vi "校准信息改变发送 (子VI).vi"(8 "错误输入":errorcluster caption="错误输出") -> (0 "错误输出":errorcluster)   [LabVIEW 2016, in "数据传输系统-04.lvlib"]
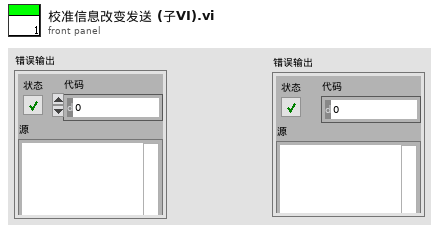
[diagram p1: front panel]
types:
  T1 = cluster{"低标液1浓度":dbl, "低标液1信号值":dbl, "低标液1启用":u16, "低标液2浓度":dbl, "低标液2信号值":dbl, "低标液2启用":u16, "低标液3浓度":dbl, "低标液3信号值":dbl, "低标液3启用":u16, "低标液4浓度":dbl, "低标液4信号值":dbl, "低标液4启用":u16, "低标液5浓度":dbl, "低标液5信号值":dbl, "低标液5启用":u16, "高标液1浓度":dbl, "高标液1信号值":dbl, "高标液1启用":u16, "高标液2浓度":dbl, "高标液2信号值":dbl, "高标液2启用":u16, "高标液3浓度":dbl, "高标液3信号值":dbl, "高标液3启用":u16, "高标液4浓度":dbl, "高标液4信号值":dbl, "高标液4启用":u16, "高标液5浓度":dbl, "高标液5信号值":dbl, "高标液5启用":u16, "低斜率":dbl, "低截距":dbl, "低二次多项式系数":dbl, "低线性相关系数":dbl, "高斜率":dbl, "高截距":dbl, "高二次多项式系数":dbl, "高线性相关系数":dbl}
  T2 = cluster{"CODMn校准信息":bool, "氨氮校准信息":bool, "总磷校准信息":bool, "总氮校准信息":bool, "CODCr校准信息":bool}
  T3 = cluster{"低标液1浓度":dbl, "低标液1信号值":dbl, "低标液1启用":u16, "低标液2浓度":dbl, "低标液2信号值":dbl, "低标液2启用":u16, "低标液3浓度":dbl, "低标液3信号值":dbl, "低标液3启用":u16, "低标液4浓度":dbl, "低标液4信号值":dbl, "低标液4启用":u16, "低标液5浓度":dbl, "低标液5信号值":dbl, "低标液5启用":u16, "高标液1浓度":dbl, "高标液1信号值":dbl, "高标液1启用":u16, "高标液2浓度":dbl, "高标液2信号值":dbl, "高标液2启用":u16, "高标液3浓度":dbl, "高标液3信号值":dbl, "高标液3启用":u16, "高标液4浓度":dbl, "高标液4信号值":dbl, "高标液4启用":u16, "高标液5浓度":dbl, "高标液5信号值":dbl, "高标液5启用":u16, "低斜率":dbl, "低截距":dbl, "低二次多项式系数":dbl, "低线性相关系数":dbl, "高斜率":dbl, "高截距":dbl, "高二次多项式系数":dbl, "高线性相关系数":dbl}[]
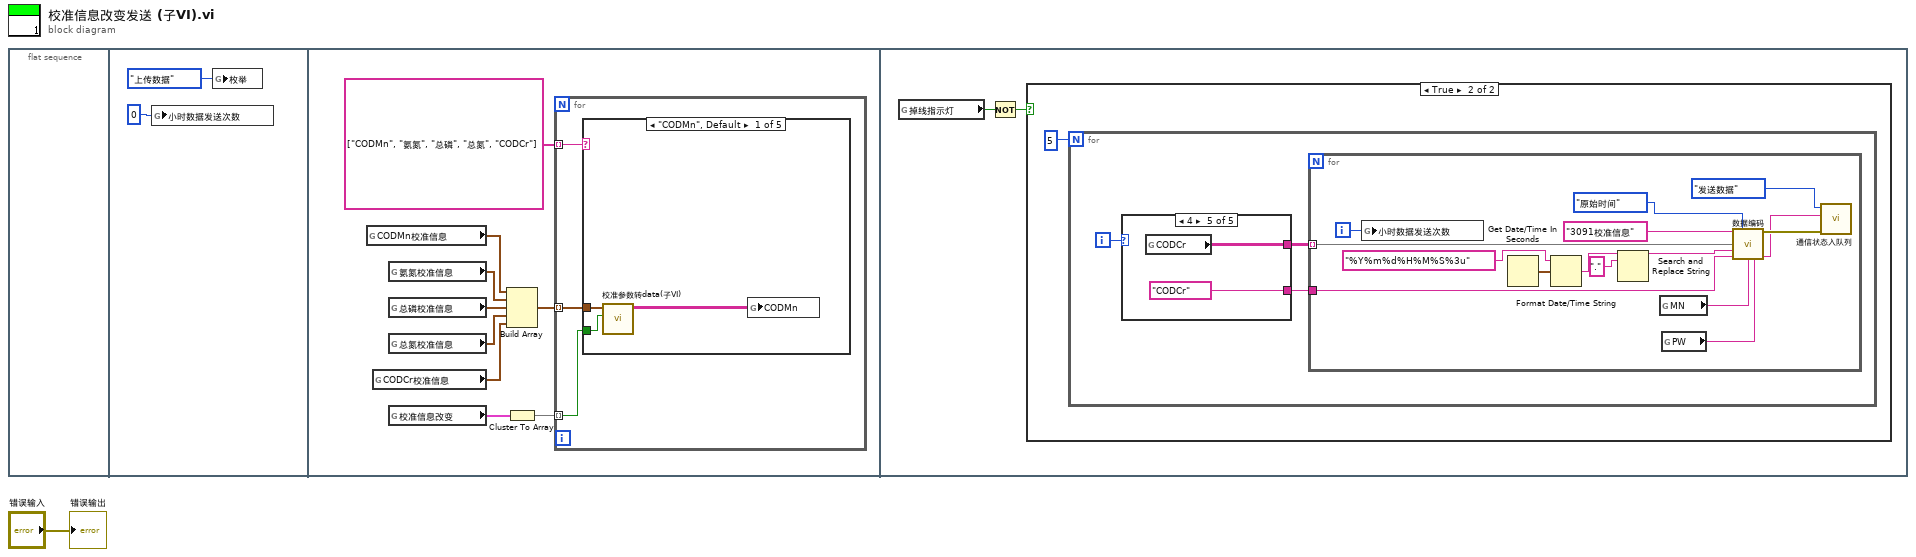
[diagram p0: block diagram]
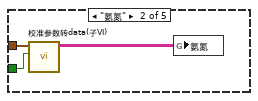
[diagram p2: hidden frame]
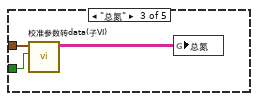
[diagram p3: hidden frame]
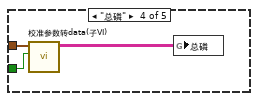
[diagram p4: hidden frame]
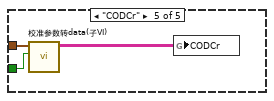
[diagram p5: hidden frame]
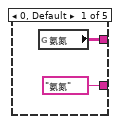
[diagram p7: hidden frame]
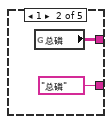
[diagram p8: hidden frame]
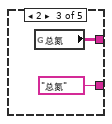
[diagram p9: hidden frame]
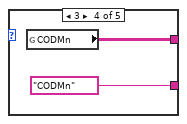
[diagram p10: hidden frame]
diagram:
  n1 = flat-sequence {
    frame #0 {
    }
    frame #1 {
      n2 = global write "全局 小时数据发送次数.vi" "小时数据发送次数"(0 ("小时数据发送次数")) -> ()
      n3 = global write "全局1.vi" "枚举"(enum16{"返回请求应答", "上传数据", "返回执行结果"}."上传数据" ("枚举")) -> ()
    }
    frame #2 {
      n4 = global read "全局1.vi" "CODMn校准信息"() -> (w9:T1)
      n5 = global read "全局1.vi" "CODCr校准信息"() -> (w12:T1)
      n6 = global read "全局1.vi" "氨氮校准信息"() -> (w11:T1)
      n7 = global read "全局1.vi" "总磷校准信息"() -> (w7:T1)
      n8 = global read "全局1.vi" "总氮校准信息"() -> (w6:T1)
      n9 = global read "全局1.vi" "校准信息改变"() -> (w5:T2)
      n10 = Build Array(w9, w11, w7, w6, w12) -> (w10:T3)
      n11 = Cluster To Array(cluster=w5) -> (array=w4:bool[])
      n12 = for {
        tunnel: string[] ["CODMn", "氨氮", "总磷", "总氮", "CODCr"] -> [w15] mode=indexing
        tunnel: w10 -> [w14] mode=indexing
        tunnel: w4 -> [w13] mode=indexing
        n13 = case shown="\"CODMn\", Default" w15 {
          tunnel: w14 -> [w18 w21 w24 w27 w30]
          tunnel: w13 -> [w17 w20 w23 w26 w29]
          frame "CODMn", Default {
            n14 = call "校准参数转data(子VI).vi"("改变?"=w17, "校准信息"=w18) -> ("数组"=w16:string[][])  [unwired: 9 in]
            n15 = global write "全局 所有参数.vi" "CODMn"(w16) -> ()
          }
          frame "氨氮" {
            n16 = call "校准参数转data(子VI).vi"("改变?"=w20, "校准信息"=w21) -> ("数组"=w19:string[][])  [unwired: 9 in]
            n17 = global write "全局 所有参数.vi" "氨氮"(w19) -> ()
          }
          frame "总氮" {
            n18 = call "校准参数转data(子VI).vi"("改变?"=w23, "校准信息"=w24) -> ("数组"=w22:string[][])  [unwired: 9 in]
            n19 = global write "全局 所有参数.vi" "总氮"(w22) -> ()
          }
          frame "总磷" {
            n20 = call "校准参数转data(子VI).vi"("改变?"=w26, "校准信息"=w27) -> ("数组"=w25:string[][])  [unwired: 9 in]
            n21 = global write "全局 所有参数.vi" "总磷"(w25) -> ()
          }
          frame "CODCr" {
            n22 = call "校准参数转data(子VI).vi"("改变?"=w29, "校准信息"=w30) -> ("数组"=w28:string[][])  [unwired: 9 in]
            n23 = global write "全局 所有参数.vi" "CODCr"(w28) -> ()
          }
        }
      }
    }
    frame #3 {
      n24 = global read "全局 数据发送重叠.vi" "掉线指示灯"() -> (w32:bool)
      n25 = Not(x=w32) -> (.not. x?=w31:bool)
      n26 = case shown="True" w31 {
        frame False {
        }
        frame True {
          n27 = for {
            N: 5 -> [_]
            i -> [w36]
            n28 = case shown="4" w36 {
              tunnel: [w38 w40 w42 w44 w46] -> w35
              tunnel: ["氨氮" ("污染物编码") "总磷" ("污染物编码") "总氮" ("污染物编码") "CODMn" ("污染物编码") "CODCr" ("污染物编码")] -> w34
              frame 0, Default {
                n29 = global read "全局 所有参数.vi" "氨氮"() -> (w38:string[][])
              }
              frame 1 {
                n30 = global read "全局 所有参数.vi" "总磷"() -> (w40:string[][])
              }
              frame 2 {
                n31 = global read "全局 所有参数.vi" "总氮"() -> (w42:string[][])
              }
              frame 3 {
                n32 = global read "全局 所有参数.vi" "CODMn"() -> (w44:string[][])
              }
              frame 4 {
                n33 = global read "全局 所有参数.vi" "CODCr"() -> (w46:string[][])
              }
            }
            n34 = for {
              tunnel: w34 -> [w61]
              tunnel: w35 -> [w60] mode=indexing
              i -> [w59]
              n35 = global write "全局 小时数据发送次数.vi" "小时数据发送次数"(w59) -> ()
              n36 = Get Date/Time In Seconds() -> (seconds since 1Jan1904=w56:timestamp)
              n37 = Format Date/Time String(time format string (%c)="%Y%m%d%H%M%S%3u" ("时间格式字符串(%c)"), seconds (now)=w56) -> (date/time string=w55:string)  [unwired: 1 in]
              n38 = Search and Replace String(input string=w55, search string="." ("搜索字符串")) -> (result string=w53:string)  [unwired: 6 in, 3 out]
              n39 = global read "断电保存全局.vi" "MN"() -> (w52:string)
              n40 = global read "断电保存全局.vi" "PW"() -> (w51:string)
              n41 = call "数据编码.vi"("table输入"="3091校准信息" ("新元素/子数组"), "仪器参数上传时间"=enum16{"精确到小时", "原始时间"}."原始时间", "仪器参数"=w60, "QN"=w53, "参数"=w61, "MN"=w52, "PW"=w51) -> ("错误常量"=w50:errorcluster, "通讯包字符串"=w47:string)  [unwired: 7 in]
              n42 = call "通信状态入队列.vi"("错误输入（无错误）"=w50, "发送报文"=w47, "枚举"=enum16{"打开连接", "发送数据", "读取数据", "数据处理", "关闭连接"}."发送数据") -> ()  [unwired: 8 in, 1 out]
            }
          }
        }
      }
    }
  }
  "错误输出" <- "错误输入"
